vi "Spin Ez.vi"(0 "Get All":T2 {"Calibration"."CurrentMode" items=["BootTareGryoAccel"=0, "Temperature"=1, "Magnetometer12Pt"=2, "Magnetometer360"=3, "Accelerometer"=5]}, 1 "Right Motor":dbl, 2 "Left Motor":dbl, 5 "Axes":dbl[](array[numeric]), 9 "Buttons":bool[](array[boolean]), 12 "P Gain":dbl=0.0725 format="%#_13g", 14 "D Gain":dbl=5e-05 format="%#_13g") -> (3 "Control Mode":T1, 4 "Right Motor Value":dbl, 6 "Left Motor Value":dbl)   [LabVIEW 2016]
doc: "When the B button is not pressed the VI sends through the motor values. When the button is pressed the direction of the robot can be controled by using the left joystick as a dial.\n\nCreated by Team 4130 for use in the 2016-2017 season"
uses:
  <vilib>/Rock Robotics/WPI/ThirdParty/Sensors/Pigeon IMU/CTRE_PigeonIMU_GlobalStatus.ctl
  <vilib>/Rock Robotics/WPI/ThirdParty/Sensors/Pigeon IMU/CTRE_PigeonIMU_PigeonState.ctl
  <vilib>/Rock Robotics/WPI/ThirdParty/Sensors/Pigeon IMU/CTRE_PigeonIMU_CalibrationMode.ctl
  <vilib>/Rock Robotics/WPI/ThirdParty/CanMotor/TalonSRX/WPI_CANTalonSRX_APIControlMode.ctl
panel:
  out "Heading":dbl(knob) scale=-360.0..360.0
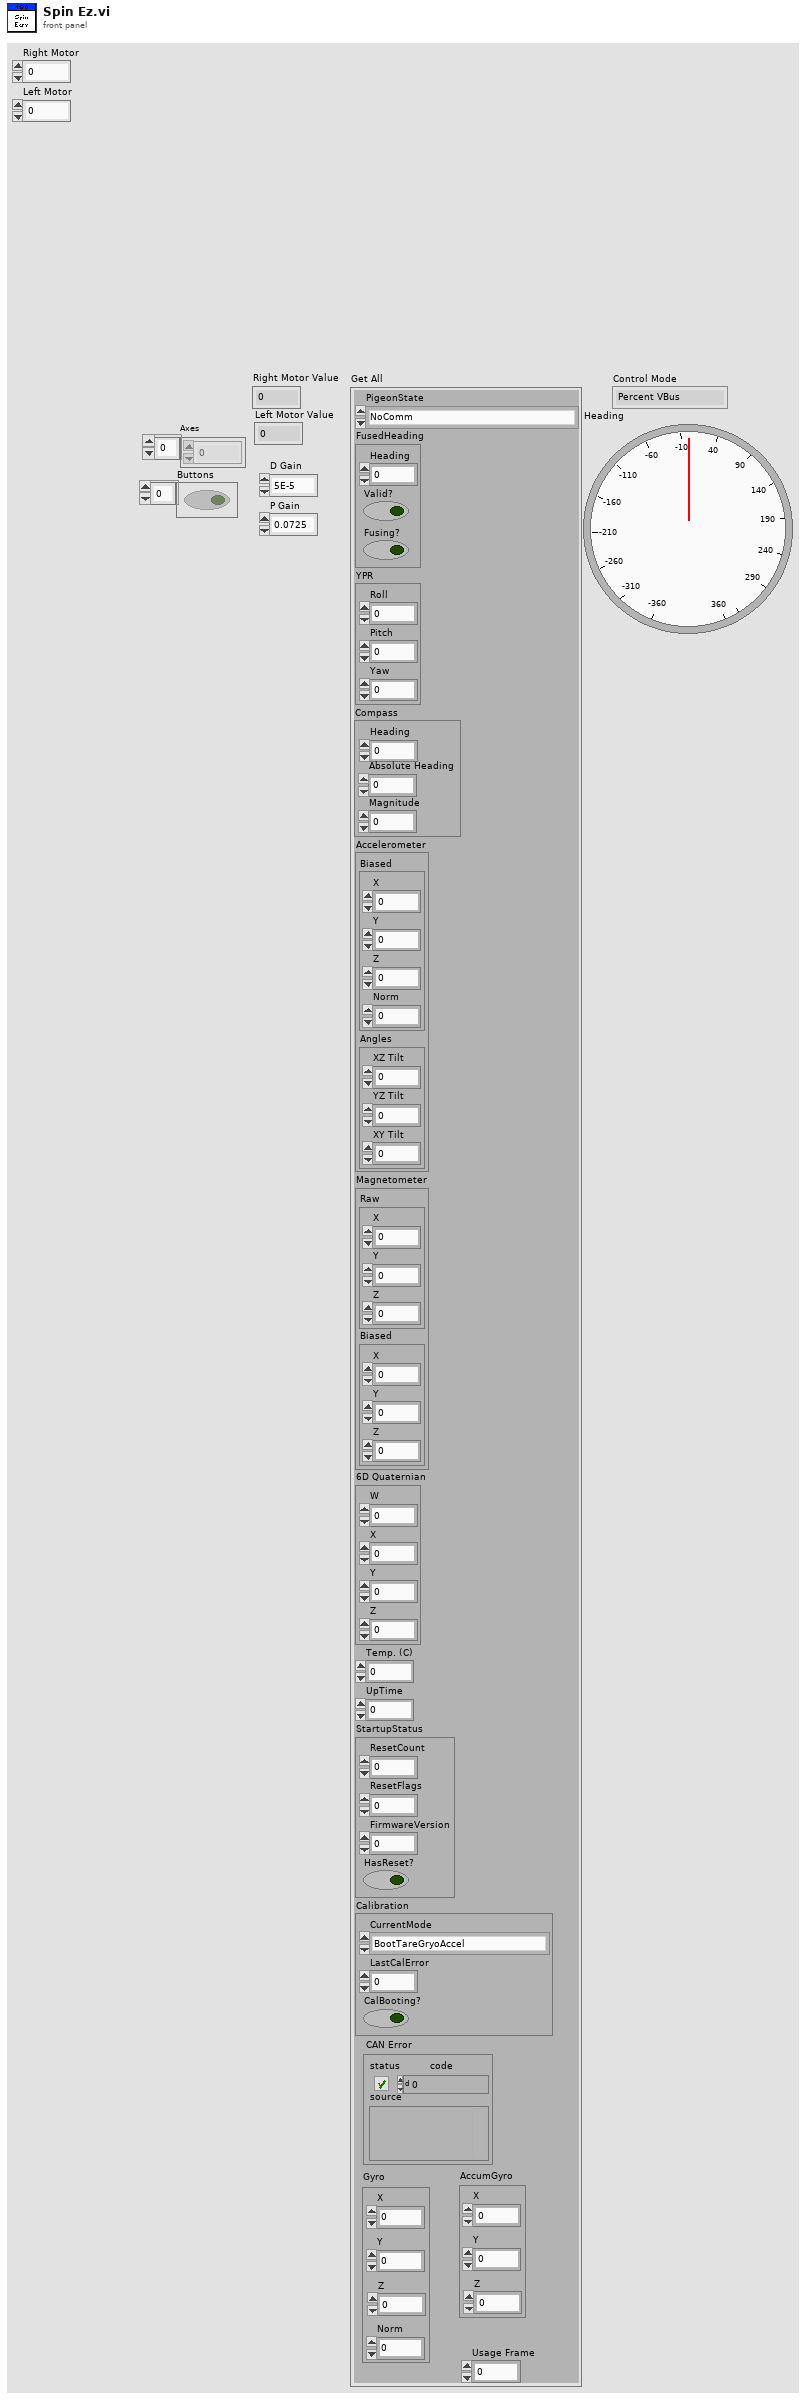
[diagram p1: front panel]
types:
  T1 = typedef "WPI_CANTalonSRX_APIControlMode.ctl" = enum8{"Percent VBus", "Speed", "Position", "Slave", "Unchanged / Invalid", "Voltage Compensation", "Current", "Motion Profile", "Motion Magic"}
  T2 = typedef "CTRE_PigeonIMU_GlobalStatus.ctl" = cluster{"PigeonState":T3, "FusedHeading":cluster{"Heading":dbl, "Valid?":bool, "Fusing?":bool}, "YPR":cluster{"Yaw":dbl, "Pitch":dbl, "Roll":dbl}, "Compass":cluster{"Heading":dbl, "Magnitude":dbl, "Absolute Heading":dbl}, "Accelerometer":cluster{"Biased":cluster{"X":i16, "Y":i16, "Z":i16, "Norm":i16}, "Angles":cluster{"XZ Tilt":dbl, "YZ Tilt":dbl, "XY Tilt":dbl}}, "Magnetometer":cluster{"Raw":cluster{"X":i16, "Y":i16, "Z":i16}, "Biased":cluster{"X":i16, "Y":i16, "Z":i16}}, "Gyro":cluster{"X":dbl, "Y":dbl, "Z":dbl, "Norm":dbl}, "6D Quaternian":cluster{"W":dbl, "X":dbl, "Y":dbl, "Z":dbl}, "Temp. (C)":dbl, "UpTime":u32, "StartupStatus":cluster{"ResetCount":i32, "ResetFlags":i32, "FirmwareVersion":i32, "HasReset?":bool}, "Calibration":cluster{"CurrentMode":T4, "LastCalError":i32, "CalBooting?":bool}, "CAN Error":errorcluster, "AccumGyro":cluster{"X":dbl, "Y":dbl, "Z":dbl}, "Usage Frame":u32}
  T3 = typedef "CTRE_PigeonIMU_PigeonState.ctl" = enum16{"NoComm", "Initializing", "Ready", "UserCalibration"}
  T4 = typedef "CTRE_PigeonIMU_CalibrationMode.ctl" = u16
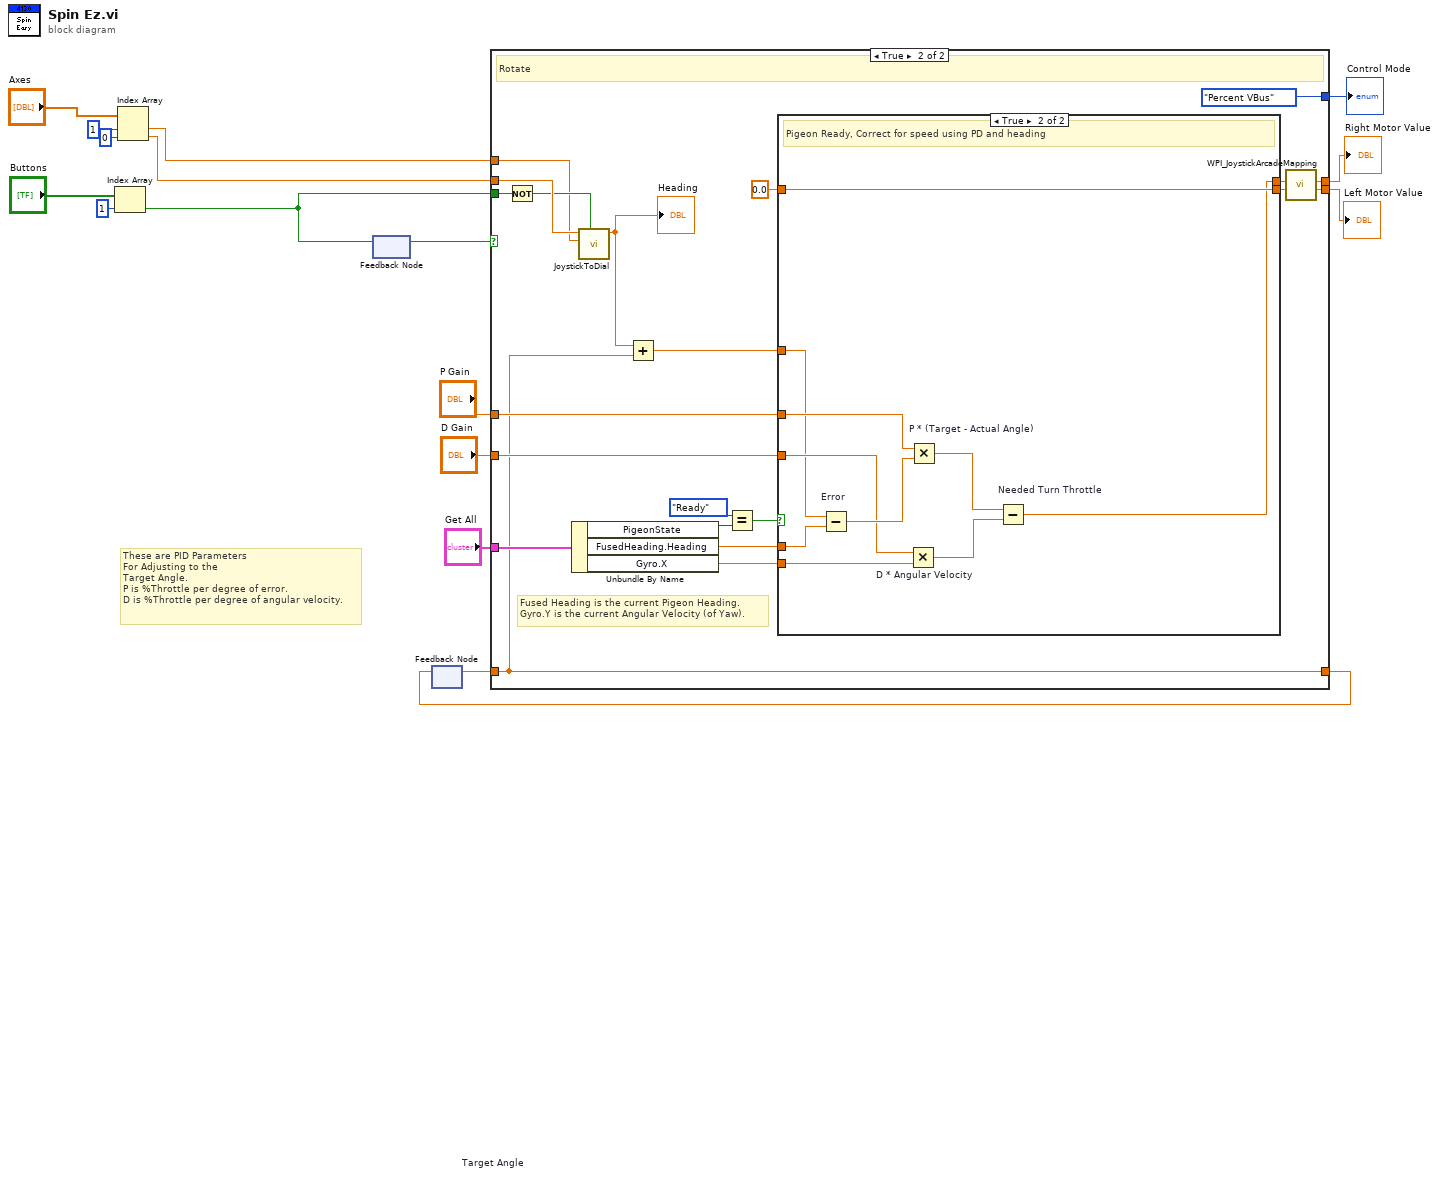
[diagram p0: block diagram]
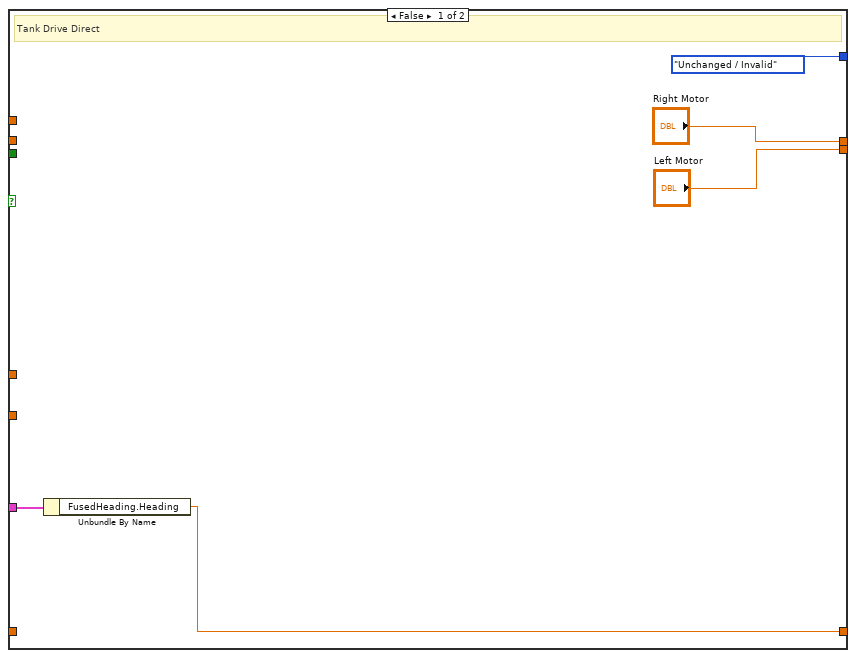
[diagram p2: hidden frame]
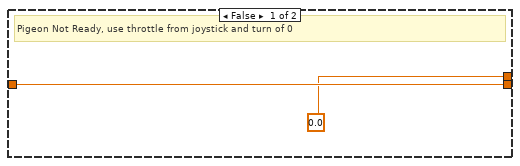
[diagram p3: hidden frame]
diagram:
  # "These are PID Parameters\nFor Adjusting to the\nTarget Angle.\nP is %Throttle per degree of error.\nD is %Throttle per degree of angular velocity."
  n1 = Index Array(array="Buttons", index=1) -> (element=w1:bool)
  n2 = Index Array(array="Axes", index #1=1 ("index"), index #2=0 ("index")) -> (element #1=w10:dbl, element #2=w6:dbl)
  n3 = feedback-in #1(w1) -> ()
  n4 = feedback #1() -> (w2:bool)  [unwired: 1 in]
  n5 = feedback #2 "Target Angle"() -> (w15:dbl)  [unwired: 1 in]
  n6 = case shown="True" w2 {
    tunnel: w10 -> [_ w24]
    tunnel: "P Gain" -> [_ w38]
    tunnel: "D Gain" -> [_ w37]
    tunnel: [w20 w29] -> w14
    tunnel: w15 -> [_ w29]
    tunnel: ["Right Motor" w34] -> w13
    tunnel: ["Left Motor" w33] -> w12
    tunnel: "Get All" -> [w22 w32]
    tunnel: [WPI_CANTalonSRX_APIControlMode."Unchanged / Invalid" ("Control Mode") WPI_CANTalonSRX_APIControlMode."Percent VBus" ("Control Mode")] -> w8
    tunnel: w6 -> [_ w27]
    tunnel: w1 -> [_ w25]
    frame False {
      # "Tank Drive Direct"
      n7 = Unbundle By Name(w22) -> ("FusedHeading.Heading"=w20:dbl)
    }
    frame True {
      # "Fused Heading is the current Pigeon Heading.\nGyro.Y is the current Angular Velocity (of Yaw)."
      # "Rotate"
      n8 = Not(x=w25) -> (.not. x?=w26:bool)
      n9 = Unbundle By Name(w32) -> ("PigeonState"=w41:T3, "FusedHeading.Heading"=w40:dbl, "Gyro.X"=w39:dbl)
      n10 = call "JoystickToDial.vi"("Reset"=w26, "Y"=w24, "X"=w27) -> ("Heading"=w30:dbl)  [unwired: 7 in, 1 out]
      "Heading" <- w30
      n11 = Add(x=w30, y=w29) -> (x+y=w28:dbl)
      n12 = Equal?(x=CTRE_PigeonIMU_PigeonState."Ready" ("PigeonState"), y=w41) -> (x = y?=w43:bool)
      n13 = case shown="True" w43 {
        tunnel: 0.0 ("upper limit") -> [w45 w48]
        tunnel: [w45 w48] -> w35
        tunnel: [0.0 ("upper limit") w46] -> w36
        tunnel: w40 -> [_ w55]
        tunnel: w28 -> [_ w47]
        tunnel: w39 -> [_ w52]
        tunnel: w38 -> [_ w53]
        tunnel: w37 -> [_ w51]
        frame False {
          # "Pigeon Not Ready, use throttle from joystick and turn of 0"
        }
        frame True {
          # "Pigeon Ready, Correct for speed using PD and heading"
          n14 = Subtract "Error"(x=w47, y=w55) -> (x-y=w54:dbl)
          n15 = Multiply "D * Angular Velocity"(x=w51, y=w52) -> (x*y=w49:dbl)
          n16 = Multiply "P * (Target - Actual Angle)"(x=w53, y=w54) -> (x*y=w50:dbl)
          n17 = Subtract "Needed Turn Throttle"(x=w50, y=w49) -> (x-y=w46:dbl)
        }
      }
      n18 = call <vilib>:"WPI_JoystickArcadeMapping.vi"("Y axis value"=w35, "X axis value"=w36) -> ("Right Motor Value"=w33:dbl, "Left Motor Value"=w34:dbl)  [unwired: 8 in]
    }
  }
  "Right Motor Value" <- w13
  "Left Motor Value" <- w12
  "Control Mode" <- w8
  n19 = feedback-in #2(w14) -> ()
